vi "Get Cluster Datatype Name.vi"(8 "error in (no error)":errorcluster, 11 "Terminal in":refnum<vi>) -> (0 "error out":errorcluster, 3 "typedef name":string)   [LabVIEW 2014]
doc: "Return Clutser datatype name.\nIf cluster is typedef. returns it's typedef name, otherwise returns autogenerated name."
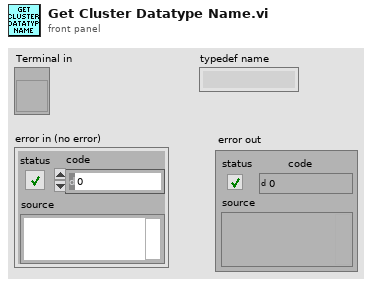
[diagram p1: front panel]
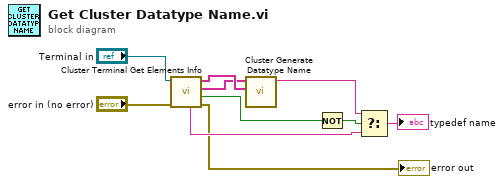
[diagram p0: block diagram]
diagram:
  n1 = call "Cluster Terminal Get Elements Info.vi"("error in (no error)"="error in (no error)", "Terminal in"="Terminal in") -> ("error out"=→"error out":errorcluster, "is typedef?"=w7:bool, "Cluster elements datatypes"=w4:string[], "Cluster elements names"=w5:string[], "typedef name"=w8:string)  [unwired: 5 in]
  n2 = call "Cluster Generate Datatype Name.vi"("Cluster elements names"=w5, "Cluster elements datatypes"=w4) -> ("generated datatype name"=w9:string)  [unwired: 9 in]
  n3 = Not(x=w7) -> (.not. x?=w6:bool)
  n4 = Select(t=w9, s=w6, f=w8) -> (s? t:f=→"typedef name":string)
